vi "direct_labview_acquire_class.vi"() -> ()   [LabVIEW 2018]
uses:
  <vilib>/Enthought/Python Integration Toolkit/api/Unpack Int.vi
panel:
  in  "Function or Method Name":string
  out "fold":bool
  out "relax":bool
  out "output":i32
  out "iteration":i32
  in  "Path to Python Module (.py File)":path=path ""
  out "Array":dbl[](array[numeric])
  out "data":dynamicdata(graph)
  in  "stop":bool
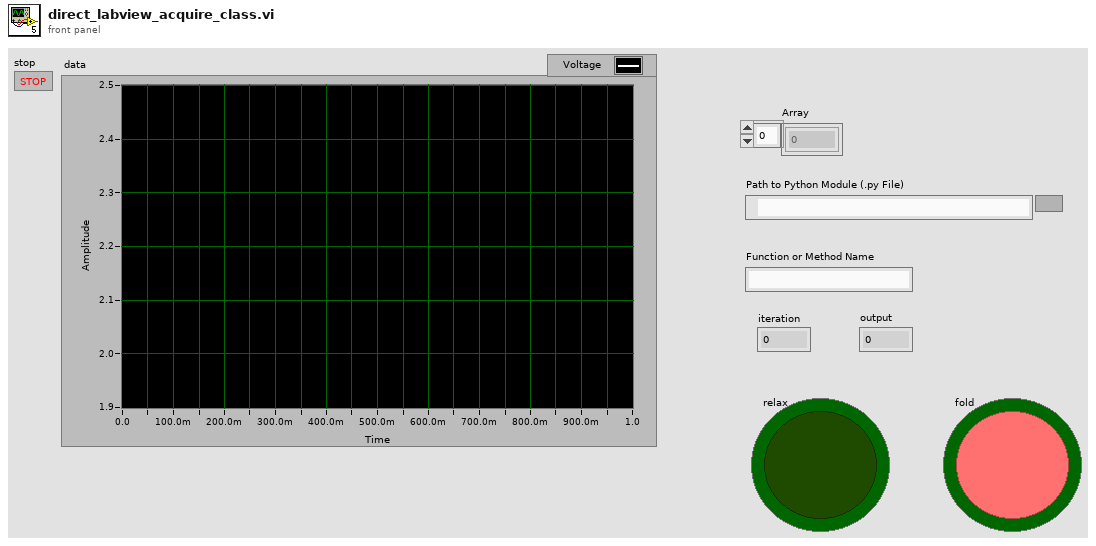
[diagram p1: front panel]
types:
  T1 = typedef "Python Integration Toolkit.lvlib/Session ID.ctl" = u64
  T2 = typedef "Python Integration Toolkit.lvlib/Python Objects.ctl" = variant
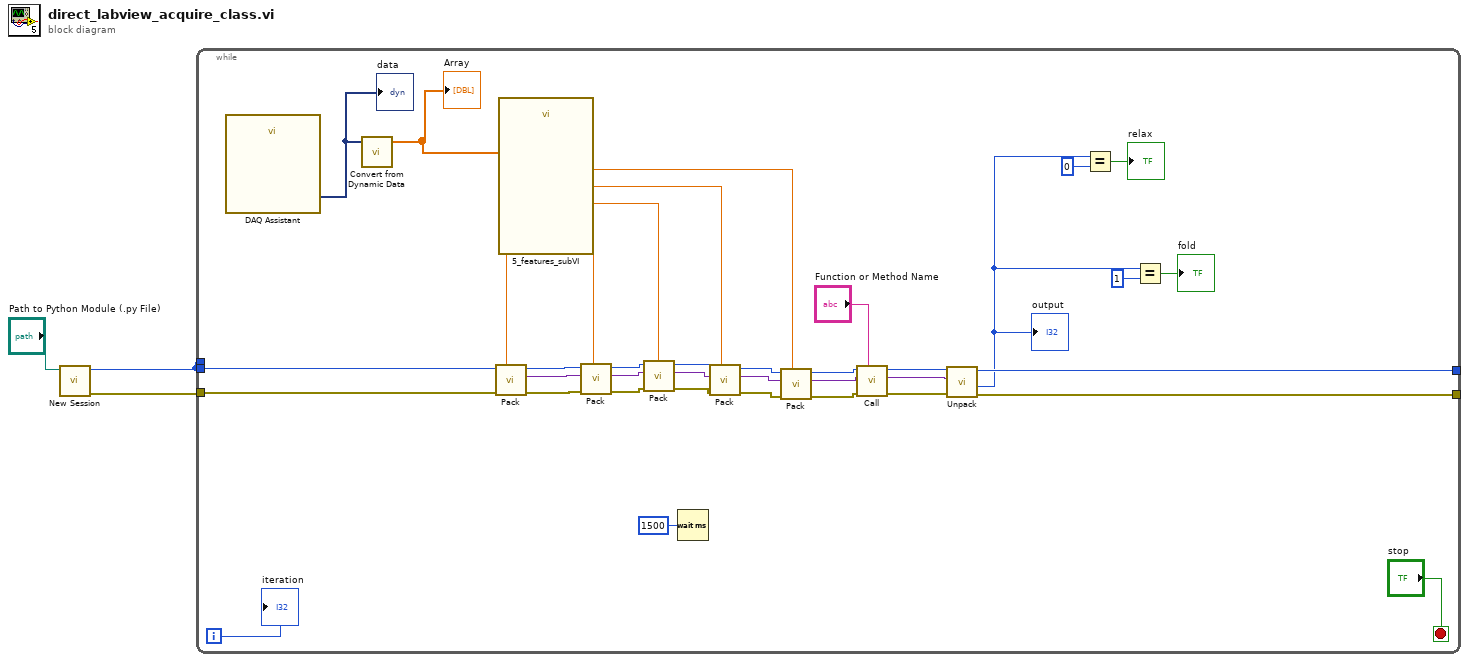
[diagram p0: block diagram]
diagram:
  n1 = call <vilib>:"New Session.vi"("Path to Python Module (.py File)"="Path to Python Module (.py File)") -> ("error out"=w2:errorcluster, "Session ID out"=w3:T1)  [unwired: 9 in]
  n2 = while {
    tunnel: w3 -> [_]
    tunnel: w3 -> [w20]
    tunnel: w2 -> [w19]
    tunnel: [w18] -> _
    tunnel: [w17] -> _
    i -> [w16]
    stop <- "stop" stop-if-true
    n3 = call "DAQ Assistant"() -> ("data"=w40:dynamicdata)  [unwired: 17 in, 2 out]
    "data" <- w40
    n4 = call "Convert from Dynamic Data"("Dynamic Data Type"=w40) -> ("Array"=w39:dbl[])  [unwired: 3 in]
    "Array" <- w39
    n5 = call "5_features_subVI.vi"("Array"=w39) -> ("skewness"=w10:dbl, "standard deviation"=w7:dbl, "mean"=w8:dbl, "kurtosis"=w9:dbl, "rms value"=w6:dbl)  [unwired: 6 in]
    n6 = call <vilib>:"Pack.vi"("Argument"=w10, "error in (no error)"=w19, "Session ID"=w20) -> ("error out"=w37:errorcluster, "Python Object References Out"=w36:T2, "Session ID out"=w38:T1)  [unwired: 6 in]
    n7 = call <vilib>:"Pack.vi"("Argument"=w9, "error in (no error)"=w37, "Python Object References In"=w36, "Session ID"=w38) -> ("error out"=w34:errorcluster, "Python Object References Out"=w33:T2, "Session ID out"=w35:T1)  [unwired: 5 in]
    n8 = call <vilib>:"Pack.vi"("Argument"=w8, "error in (no error)"=w34, "Python Object References In"=w33, "Session ID"=w35) -> ("error out"=w31:errorcluster, "Python Object References Out"=w30:T2, "Session ID out"=w32:T1)  [unwired: 5 in]
    n9 = Wait (ms)(milliseconds to wait=u32 1500) -> ()  [unwired: 1 out]
    n10 = call <vilib>:"Pack.vi"("Argument"=w7, "error in (no error)"=w31, "Python Object References In"=w30, "Session ID"=w32) -> ("error out"=w28:errorcluster, "Python Object References Out"=w27:T2, "Session ID out"=w29:T1)  [unwired: 5 in]
    n11 = call <vilib>:"Pack.vi"("Argument"=w6, "error in (no error)"=w28, "Python Object References In"=w27, "Session ID"=w29) -> ("error out"=w25:errorcluster, "Python Object References Out"=w24:T2, "Session ID out"=w26:T1)  [unwired: 5 in]
    n12 = call <vilib>:"Call.vi"("Function or Method Name"="Function or Method Name", "error in (no error)"=w25, "Python Object References In"=w24, "Session ID"=w26) -> ("error out"=w22:errorcluster, "Python Object References Out"=w21:T2, "Session ID out"=w23:T1)  [unwired: 5 in]
    n13 = call-poly <vilib>:"Unpack.vi"("error in (no error)"=w22, "Python Object References In"=w21, "Session ID"=w23) -> ("error out"=w17:errorcluster, "Value"=w14:i32, "Session ID out"=w18:T1)  [unwired: 5 in, 1 out]
    "output" <- w14
    n14 = Equal?(x=w14, y=0) -> (x = y?=→"relax":bool)
    n15 = Equal?(x=w14, y=1) -> (x = y?=→"fold":bool)
    "iteration" <- w16
  }
